vi "loadGraph(SubVI).vi"() -> (1 "String":string, 2 "all rows":dbl[][](array[numeric]))   [LabVIEW 2025]
uses:
  <vilib>/Utility/file.llb/Read Delimited Spreadsheet (DBL).vi
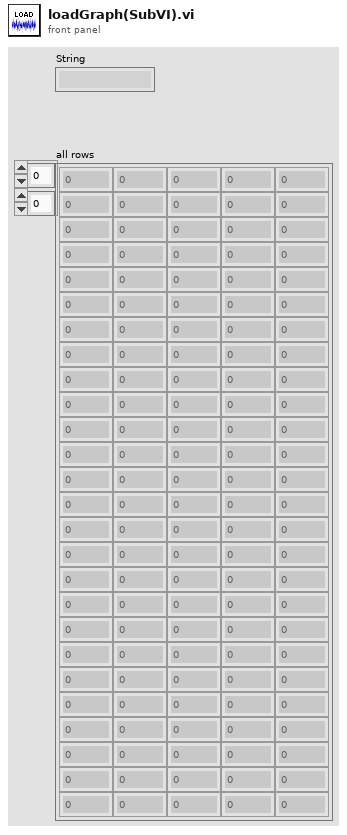
[diagram p1: front panel]
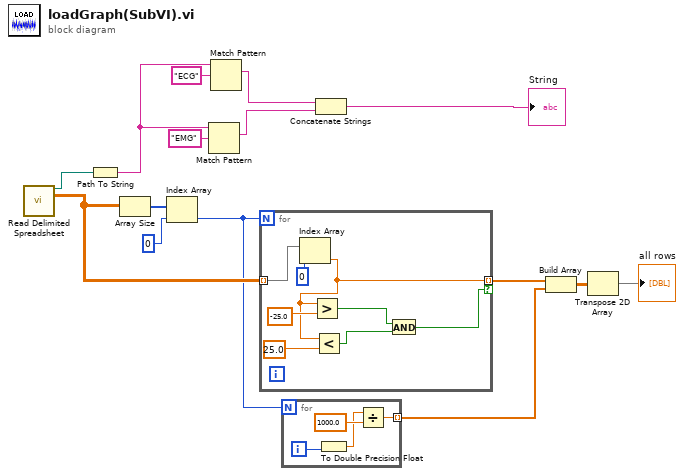
[diagram p0: block diagram]
diagram:
  n1 = call-poly <vilib>:"Read Delimited Spreadsheet.vi"() -> ("new file path (Not A Path if cancelled)"=w15:path, "all rows"=w12:dbl[][])  [unwired: 10 in, 4 out]
  n2 = Path To String(path=w15) -> (string=w5:string)
  n3 = Array Size(array=w12) -> (size(s)=w13:i32[])
  n4 = Index Array(array=w13, index=0) -> (element=w11:i32)
  n5 = Match Pattern(string=w5, regular expression="EMG") -> (match substring=w2:string)  [unwired: 1 in, 3 out]
  n6 = Match Pattern(string=w5, regular expression="ECG") -> (match substring=w3:string)  [unwired: 1 in, 3 out]
  n7 = for {
    N: w11 -> [_]
    tunnel: w12 -> [w21] mode=indexing
    tunnel: [w19] -> w9 mode=indexing if=w16
    n8 = Index Array(array=w21, index=0) -> (element=w19:dbl)
    n9 = Greater?(x=w19, y=-25.0) -> (0:w18:bool)
    n10 = Less?(x=w19, y=25.0) -> (x < y?=w17:bool)
    n11 = And(x=w18, y=w17) -> (x .and. y?=w16:bool)
  }
  n12 = for {
    N: w11 -> [_]
    tunnel: [w24] -> w10 mode=indexing
    i -> [w26]
    n13 = To Double Precision Float(number=w26) -> (double precision float=w25:dbl)
    n14 = Divide(x=w25, y=1000.0) -> (x/y=w24:dbl)
  }
  n15 = Concatenate Strings(w3, w2) -> (→"String":string)
  n16 = Build Array(w9, w10) -> (w8:dbl[][])
  n17 = Transpose 2D Array(2D array=w8) -> (transposed array=→"all rows":dbl[][])
